vi "GetBaseLineOffset.vi"(3 "error in (no error)":errorcluster, 4 "Return Parameter":u8(ring) items=["Value", "Minimum", "Maximum"], 5 "Channel (0: Channel 1)":u16(ring) items=["Channel 1", "Channel 2", "Channel 3", "Channel 4", "Channel 5", "Channel 6", "Channel 7", "Channel 8"], 6 "VISA resource name":refnum<visa-resource-name>) -> (0 "error out":errorcluster, 1 "Base Line Offset (V)":dbl format="%#_16g", 2 "VISA resource name out":refnum<visa-resource-name>)   [LabVIEW 2020, in "Active Technologies AWG3000.lvlib"]
uses:
  Active Technologies AWG3000.lvlib
panel:
  out "read buffer":string
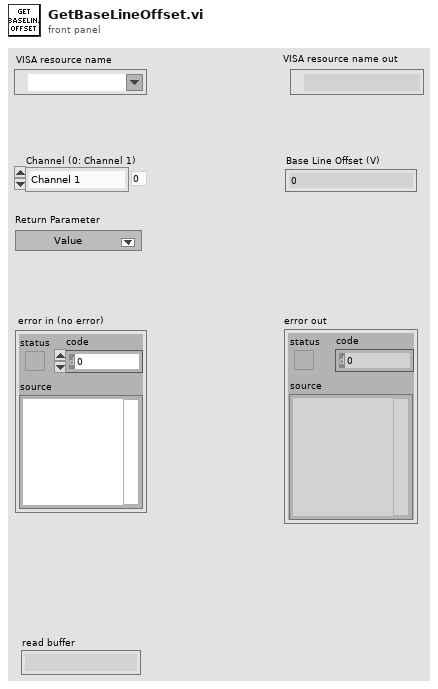
[diagram p1: front panel]
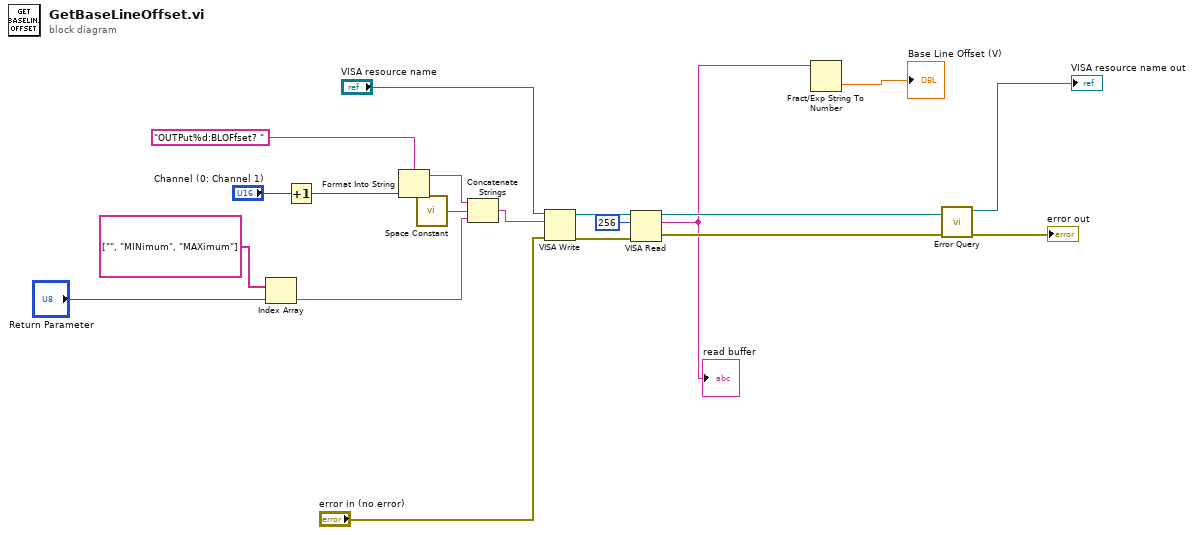
[diagram p0: block diagram]
diagram:
  n1 = Index Array(array=string[] ["", "MINimum", "MAXimum"], index="Return Parameter") -> (element=w4:string)
  n2 = Increment(x="Channel (0: Channel 1)") -> (x+1=w16:u16)
  n3 = Format Into String(format string="OUTPut%d:BLOFfset? " ("write buffer"), w16) -> (resulting string=w13:string)  [unwired: 2 in, 1 out]
  n4 = call <vilib>:"Space Constant.vi"() -> ("String"=w3:string)
  n5 = Concatenate Strings(w13, w3, w4) -> (w12:string)
  n6 = VISA Write(VISA resource name="VISA resource name", write buffer=w12, error in (no error)="error in (no error)") -> (VISA resource name out=w11:refnum<visa-resource-name>, error out=w10:errorcluster)  [unwired: 1 out]
  n7 = VISA Read(VISA resource name=w11, byte count=u32 256, error in (no error)=w10) -> (VISA resource name out=w8:refnum<visa-resource-name>, read buffer=w1:string, error out=w7:errorcluster)  [unwired: 1 out]
  "read buffer" <- w1
  n8 = Fract/Exp String To Number(string=w1) -> (number=→"Base Line Offset (V)":dbl)  [unwired: 3 in, 1 out]
  n9 = call "Error Query.vi"("error in (no error)"=w7, "VISA resource name"=w8) -> ("error out"=→"error out":errorcluster, "VISA resource name out"=→"VISA resource name out":refnum<visa-resource-name>)  [unwired: 6 in, 2 out]
